vi "Initialize.vi"(8 "error in (no error)":errorcluster, 11 "SDK Directory Path":path) -> (0 "error out":errorcluster, 3 "Result":i32)   [LabVIEW 2018, in "Fujifilm X Series GFX System Digital Camera.lvlib"]
doc: "Establishes communication with the instrument and optionally performs an instrument identification query and/or an instrument reset. It also places the instrument in a default state needed for other instrument driver operations. Therefore, call this VI before calling other instrument driver VIs for this instrument. Generally, you need to call the Initialize VI only once at the beginning of an application."
uses:
  <instrlib>/Fujifilm X Series GFX System Digital Camera/Fujifilm X Series GFX System Digital Camera.lvlib
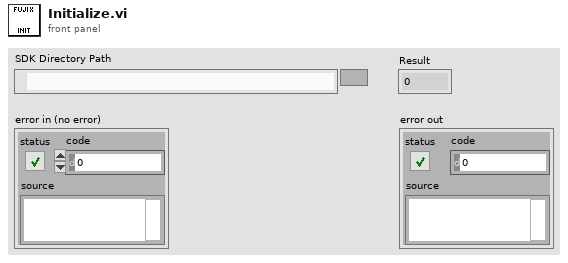
[diagram p1: front panel]
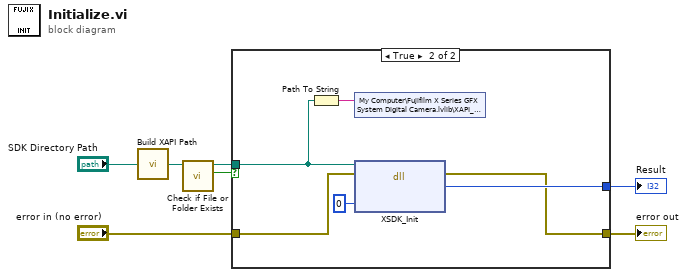
[diagram p0: block diagram]
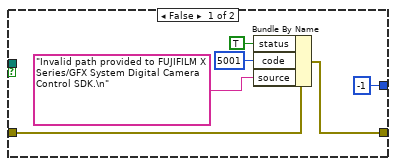
[diagram p2: hidden frame]
diagram:
  n1 = call <instrlib>:"Build XAPI Path.vi"("SDK Directory Path"="SDK Directory Path") -> ("XAPI Library Path"=w4:path)
  n2 = call <vilib>:"Check if File or Folder Exists.vi"("path"=w4) -> ("file or folder exists?"=w2:bool, "dup path"=w3:path)  [unwired: 8 in, 1 out]
  n3 = case shown="True" w2 {
    tunnel: "error in (no error)" -> [w12 w18]
    tunnel: [-1 ("result") w16] -> w6
    tunnel: [w11 w15] -> w5
    tunnel: w3 -> [_ w14]
    frame False {
      n4 = Bundle By Name(cluster=w12, "status"=TRUE, "code"=5001, "source"="Invalid path provided to FUJIFILM X Series/GFX System Digital Camera Control SDK.\n") -> (w11:errorcluster)
    }
    frame True {
      n5 = Path To String(path=w14) -> (string=w19:string)
      n6 = shared-variable "My Computer\\Fujifilm X Series GFX System Digital Camera.lvlib\\XAPI_SDK_PATH"(w19) -> ()  [unwired: 1 in, 1 out]
      n7 = dll-call lib="?" fn="XSDK_Init"(path in=w14, error in=w18, "hLib"=0) -> (error out=w15:errorcluster, "result"=w16:i32)  [unwired: 2 in, 1 out]
    }
  }
  "error out" <- w5
  "Result" <- w6
